vi "DFD FXP Set Quantizer (One).vi"(8 "error in (no error)":errorcluster, 10 "quantizer":T1={"source"=0, "wl"=16, "iwl"=1, "overflow mode"=enum."Wrap", "rounding mode"=enum."Truncation", "signed?"=TRUE} {"source" items=["Coefficients a/k"=0, "Coefficients b/v"=7, "Input"=1, "Output"=2, "Multiplicand"=3, "Product"=4, "Sum"=5, "Delay"=6]}, 11 "filter in":T3={"mSRate_Fs"=1.0, "mSRate_Version"="2.0", "mSRate_Comments"="", "mSRate_OrgCoef"={"type"=enum."Undefined", "gain"=1.0, "coef a (k)"=[], "coef b (v)"=[]}, "mSRate_CurCoef"={"type"=enum."Undefined", "gain"=1.0, "coef a (k)"=[], "coef b (v)"=[]}, "mSRate_Quantized?"=FALSE, "mSRate_QCoef"={"type"=enum."Undefined", "gain"=1.0, "coef a (k)"=[], "coef b (v)"=[]}, "mSRate_QSettings"=[], "mSRate_Order"=0, "mSRate_Scaling"={"mSRate_ScaleByPowerOf2?"=FALSE, "mSRate_ScaleType"=enum."No Norm"}} {"mSRate_QSettings"."source" items=["Coef a/k"=0, "Coef b/v"=7, "Input"=1, "Output"=2, "Multiplicand"=3, "Product"=4, "Sum"=5, "Delay"=6, "Gain"=8]}) -> (0 "error out":errorcluster, 3 "filter out":T3={"mSRate_Fs"=1.0, "mSRate_Version"="2.0", "mSRate_Comments"="", "mSRate_OrgCoef"={"type"=enum."Undefined", "gain"=1.0, "coef a (k)"=[], "coef b (v)"=[]}, "mSRate_CurCoef"={"type"=enum."Undefined", "gain"=1.0, "coef a (k)"=[], "coef b (v)"=[]}, "mSRate_Quantized?"=FALSE, "mSRate_QCoef"={"type"=enum."Undefined", "gain"=1.0, "coef a (k)"=[], "coef b (v)"=[]}, "mSRate_QSettings"=[], "mSRate_Order"=0, "mSRate_Scaling"={"mSRate_ScaleByPowerOf2?"=FALSE, "mSRate_ScaleType"=enum."No Norm"}} {"mSRate_QSettings"."source" items=["Coef a/k"=0, "Coef b/v"=7, "Input"=1, "Output"=2, "Multiplicand"=3, "Product"=4, "Sum"=5, "Delay"=6, "Gain"=8]})   [LabVIEW 2017, in "NI_DigFilterLicensed.lvlib"]
doc: "Sets a quantizer or quantizers in a fixed-point filter. You must manually select the polymorphic instance you want to use."
uses:
  <vilib>/addons/Digital Filter Design/NI_DigFilterLicensed.lvlib
  <vilib>/addons/Digital Filter Design/_Objects.llb/DFD Filter Obj.ctl
  <vilib>/addons/Digital Filter Design/_Objects.llb/DFD Filter Coef.ctl
  <vilib>/addons/Digital Filter Design/_Objects.llb/DFD Filter Structure Type Selector.ctl
  <vilib>/addons/Digital Filter Design/_Objects.llb/dfd_Internal Quantization Settings.ctl
  <vilib>/addons/Digital Filter Design/_Objects.llb/dfd_Internal Quantization Srcs.ctl
  <vilib>/addons/Digital Filter Design/_Objects.llb/DFD Coef Norm Type.ctl
  <vilib>/addons/Digital Filter Design/_Objects.llb/DFD Quantization Settings.ctl
  <vilib>/addons/Digital Filter Design/_Objects.llb/DFD Quantization Sources.ctl
  <vilib>/addons/Digital Filter Design/FXPModel.llb/DFD FXP Quantize Coef (Advanced).vi
  <vilib>/addons/Digital Filter Design/NI_DigFilter_FXP.lvlib
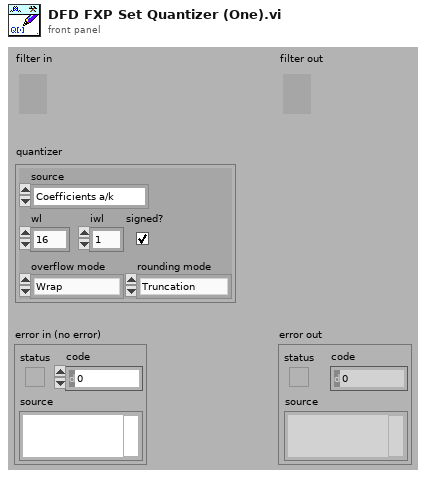
[diagram p1: front panel]
types:
  T1 = typedef "NI_DigFilterLicensed.lvlib/DFD Quantization Settings.ctl" = cluster{"source":T2, "wl":i16, "iwl":i16, "overflow mode":enum16{"Saturation", "Wrap"}, "rounding mode":enum16{"Nearest", "Truncation"}, "signed?":bool}
  T2 = typedef "NI_DigFilterLicensed.lvlib/DFD Quantization Sources.ctl" = u16
  T3 = typedef "NI_DigFilterLicensed.lvlib/DFD Filter Obj.ctl" = cluster{"mSRate_Fs":dbl, "mSRate_Version":string, "mSRate_Comments":string, "mSRate_OrgCoef":T4, "mSRate_CurCoef":T4, "mSRate_Quantized?":bool, "mSRate_QCoef":T4, "mSRate_QSettings":T6[], "mSRate_Order":i32, "mSRate_Scaling":cluster{"mSRate_ScaleByPowerOf2?":bool, "mSRate_ScaleType":T8}}
  T4 = typedef "NI_DigFilterLicensed.lvlib/DFD Filter Coef.ctl" = cluster{"type":T5, "gain":dbl, "coef a (k)":dbl[], "coef b (v)":dbl[]}
  T5 = typedef "NI_DigFilterLicensed.lvlib/DFD Filter Structure Type Selector.ctl" = enum16{"Undefined", "FIR Direct Form", "FIR Direct Form Transposed", "FIR Symmetric", "FIR Antisymmetric", "IIR Direct Form I", "IIR Direct Form I Transposed", "IIR Direct Form II", "IIR Direct Form II Transposed", "IIR Cascaded Second Order Sections Form I", "IIR Cascaded Second Order Sections Form I Transposed", "IIR Cascaded Second Order Sections Form II", "IIR Cascaded Second Order Sections Form II Transposed", "Lattice Allpass (basic sections)", "Lattice Allpass (one multiplier sections)", "Lattice Allpass (normalized sections)", "Lattice AR (basic sections)", "Lattice AR (one multiplier sections)", "Lattice AR (normalized sections)", "Lattice MA (minimum phase)", "Lattice MA (maximum phase)", "Lattice ARMA (basic sections)", "Lattice ARMA (one multiplier sections)", "Lattice ARMA (normalized sections)"}
  T6 = typedef "NI_DigFilterLicensed.lvlib/dfd_Internal Quantization Settings.ctl" = cluster{"source":T7, "wl":i16, "iwl":i16, "overflow mode":enum16{"Saturation", "Wrap"}, "rounding mode":enum16{"Nearest", "Truncation"}, "signed?":bool}
  T7 = typedef "NI_DigFilterLicensed.lvlib/dfd_Internal Quantization Srcs.ctl" = u16
  T8 = typedef "NI_DigFilterLicensed.lvlib/DFD Coef Norm Type.ctl" = enum16{"No Norm", "Time Domain 1-Norm", "Time Domain 2-Norm", "Time Domain Inf-Norm"}
  T9 = cluster{"gain processing target":u16, "gain wl":i16}
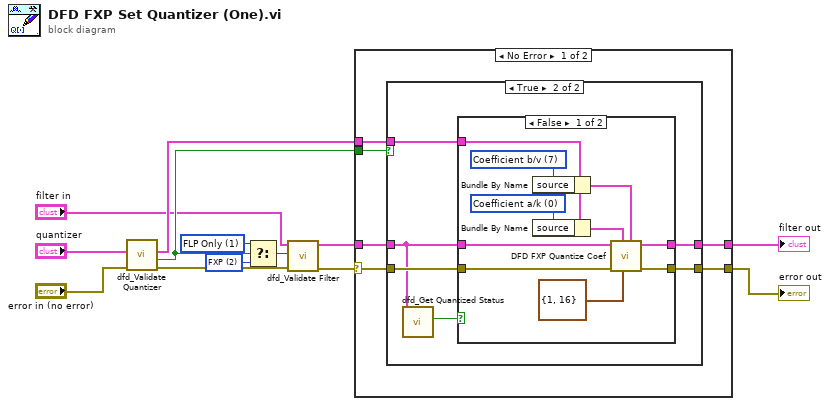
[diagram p0: block diagram]
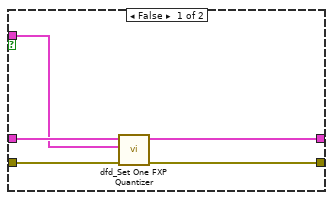
[diagram p2: hidden frame]
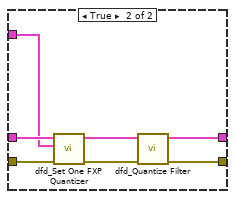
[diagram p3: hidden frame]
diagram:
  w5 = u16 2 items=["Auto", "FLP Only", "FXP"] ("check option")
  w6 = u16 1 items=["Auto", "FLP Only", "FXP"] ("check option")
  n1 = call <vilib>:"dfd_Validate Quantizer.vi"("error in (no error)"="error in (no error)", "quantizer in"="quantizer") -> ("error out"=w10:errorcluster, "coef source?"=w7:bool, "dup quantizer"=w9:T6)  [unwired: 7 out]
  n2 = Select(t=w6, s=w7, f=w5) -> (s? t:f=w4:u16)
  n3 = call <vilib>:"dfd_Validate Filter.vi"("error in (no error)"=w10, "check option"=w4, "filter in"="filter in") -> ("error out"=w2:errorcluster, "filter out"=w3:T3)  [unwired: 7 out]
  n4 = case shown="No Error" w2 {
    selector: w2 -> [w14 w48]
    tunnel: [w19 _] -> w13
    tunnel: [w18 w48] -> w12
    tunnel: w9 -> [w17 _]
    tunnel: w7 -> [w16 _]
    tunnel: w3 -> [w15 _]
    frame No Error {
      n5 = case shown="True" w16 {
        tunnel: w15 -> [w24 w26]
        tunnel: w14 -> [w23 w30]
        tunnel: w17 -> [w20 w29]
        tunnel: [w22 w28] -> w19
        tunnel: [w21 w27] -> w18
        frame False {
          n6 = call <vilib>:"dfd_Set One FXP Quantizer.vi"("error in (no error)"=w23, "quantization settings"=w20, "filter in"=w24) -> ("error out"=w21:errorcluster, "filter out"=w22:T3)  [unwired: 7 out]
        }
        frame True {
          n7 = call <vilib>:"dfd_Get Quantized Status.vi"("filter in"=w26) -> ("quantized?"=w25:bool)  [unwired: 1 in, 9 out]
          n8 = case shown="False" w25 {
            tunnel: w26 -> [w37 w45]
            tunnel: w30 -> [w36 w44]
            tunnel: w29 -> [w38 w41]
            tunnel: [w34 w47] -> w28
            tunnel: [w35 w46] -> w27
            frame False {
              w39 = T2 7 items=["Coefficient a/k"=0, "Coefficient b/v"=7, "Input"=1, "Output"=2, "Multiplicand"=3, "Product"=4, "Sum"=5, "Delay"=6] ("source")
              w40 = T2 0 items=["Coefficient a/k"=0, "Coefficient b/v"=7, "Input"=1, "Output"=2, "Multiplicand"=3, "Product"=4, "Sum"=5, "Delay"=6] ("source")
              n9 = Bundle By Name(cluster=w38, "source"=w39) -> (w32:T6)
              n10 = Bundle By Name(cluster=w38, "source"=w40) -> (w33:T6)
              n11 = call-poly <vilib>:"DFD FXP Quantize Coef.vi"("coefficients b/v quantizer"=w32, "gain settings"=T9 {"gain processing target"=1, "gain wl"=16} ("gain setting"), "coefficients a/k quantizer"=w33, "error in (no error)"=w36, "filter in"=w37) -> ("error out"=w35:errorcluster, "filter out"=w34:T3)  [unwired: 5 out]
            }
            frame True {
              n12 = call <vilib>:"dfd_Set One FXP Quantizer.vi"("error in (no error)"=w44, "quantization settings"=w41, "filter in"=w45) -> ("error out"=w43:errorcluster, "filter out"=w42:T3)  [unwired: 7 out]
              n13 = call <vilib>:"dfd_Quantize Filter.vi"("error in (no error)"=w43, "filter in"=w42) -> ("error out"=w46:errorcluster, "filter out"=w47:T3)  [unwired: 8 out]
            }
          }
        }
      }
    }
    frame Error {
    }
  }
  "filter out" <- w13
  "error out" <- w12
